vi "Write Typedef Description (path).vi"(8 "error in (no error)":errorcluster, 9 "ctl path":path, 10 "VI Description in":string) -> (0 "error out":errorcluster, 2 "VI Description out":string)   [LabVIEW 2019, in "JSON-Schema.lvlib"]
uses:
  JSON-Schema.lvlib
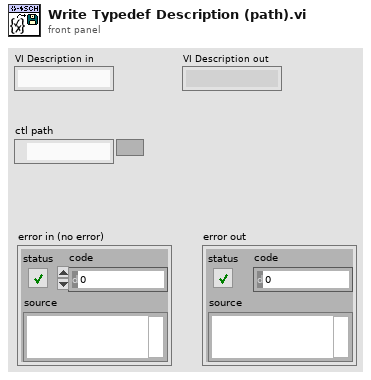
[diagram p1: front panel]
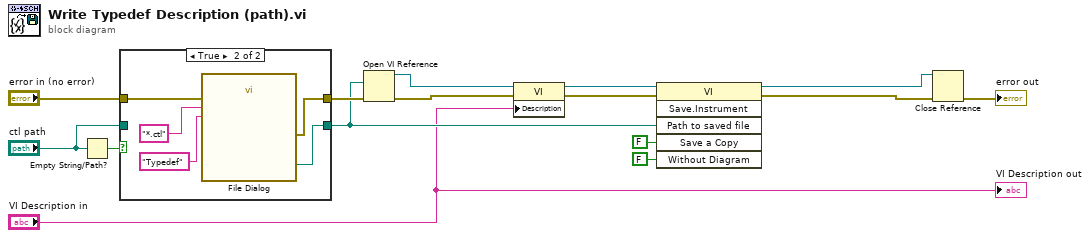
[diagram p0: block diagram]
diagram:
  n1 = Empty String/Path?(string/path="ctl path") -> (empty?=w11:bool)
  n2 = case shown="True" w11 {
    tunnel: [w17 w22] -> w7
    tunnel: "error in (no error)" -> [w16 w21]
    tunnel: [w16 w20] -> w12
    tunnel: "ctl path" -> [w17 _]
    frame False {
    }
    frame True {
      n3 = call "File Dialog"("error in"=w21, "pattern (all files)"="*.ctl", "pattern label"="Typedef") -> ("selected path"=w22:path, "error out"=w20:errorcluster)  [unwired: 9 in, 2 out]
    }
  }
  n4 = Open VI Reference(vi path=w7, error in (no error)=w12) -> (vi reference=w15:refnum<vi>, error out=w14:errorcluster)  [unwired: 4 in]
  n5 = property class="VI"(reference=w15, error in=w14, "Description"="VI Description in") -> (reference out=w5:refnum<vi>, error out=w4:errorcluster)
  n6 = invoke class="VI" method="Save.Instrument"(reference=w5, error in=w4, "Path to saved file"=w7, "Save a Copy"=FALSE, "Without Diagram"=FALSE) -> (reference out=w10:refnum<vi>, error out=w8:errorcluster)  [unwired: 1 in, 4 out]
  n7 = Close Reference(reference=w10, error in (no error)=w8) -> (error out=→"error out":errorcluster)
  "VI Description out" <- "VI Description in"
